vi "CounterStuff.vi"() -> ()   [LabVIEW 2012]
uses:
  <vilib>/DAQmx/write.llb/DAQmx Write (Analog 1D DBL 1Chan NSamp).vi
  <vilib>/DAQmx/create/channels.llb/DAQmx Create Channel (CO-Pulse Generation-Frequency).vi
  <vilib>/DAQmx/create/channels.llb/DAQmx Create Channel (AO-Voltage-Basic).vi
  <vilib>/DAQmx/configure/timing.llb/DAQmx Timing (Sample Clock).vi
  <vilib>/DAQmx/miscellaneous.llb/DAQmx Fill In Error Info.vi
panel:
  in  "stop":bool
  in  "Pixels (Lines)":dbl=256.0
  in  "Pixeltime (ms)":dbl=1.0
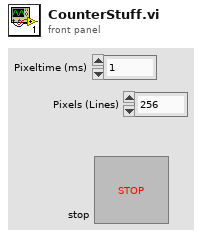
[diagram p1: front panel]
types:
  T1 = cluster{"task out":refnum<k21>, "task out":refnum<k21>, "task out":refnum<k21>, "task out":refnum<k21>}
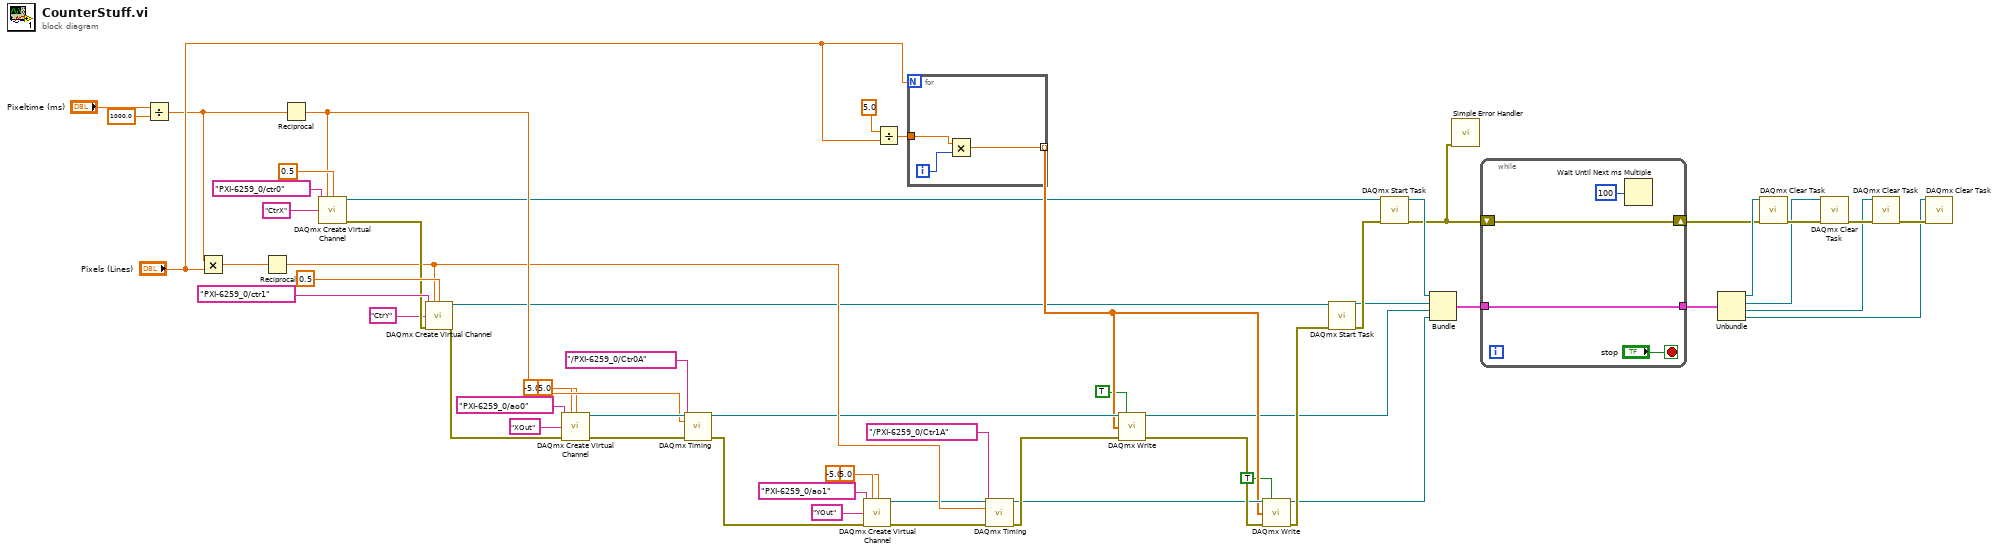
[diagram p0: block diagram]
diagram:
  n1 = Divide(x="Pixeltime (ms)", y=1000.0) -> (x/y=w7:dbl)
  n2 = Multiply(x=w7, y="Pixels (Lines)") -> (x*y=w55:dbl)
  n3 = Reciprocal(x=w55) -> (1/x=w42:dbl)
  n4 = Reciprocal(x=w7) -> (1/x=w47:dbl)
  n5 = call-poly <vilib>:"DAQmx Create Virtual Channel.vi"("frequency"=w47, "duty cycle"=0.5, "counter"=tag "PXI-6259_0/ctr0", "name to assign"="CtrX") -> ("task out"=w23:refnum<k21>, "error out"=w48:errorcluster)  [unwired: 10 in]
  n6 = call-poly <vilib>:"DAQmx Create Virtual Channel.vi"("frequency"=w42, "duty cycle"=0.5, "counter"=tag "PXI-6259_0/ctr1", "name to assign"="CtrY", "error in"=w48) -> ("task out"=w25:refnum<k21>, "error out"=w49:errorcluster)  [unwired: 9 in]
  n7 = call-poly <vilib>:"DAQmx Create Virtual Channel.vi"("maximum value"=5.0, "minimum value"=-5.0, "physical channels"=tag "PXI-6259_0/ao0", "name to assign"="XOut", "error in"=w49) -> ("task out"=w51:refnum<k21>, "error out"=w52:errorcluster)  [unwired: 9 in]
  n8 = call-poly <vilib>:"DAQmx Timing.vi"("task/channels in"=w51, "rate"=w47, "source"=tag "/PXI-6259_0/Ctr0A", "error in"=w52) -> ("task out"=w40:refnum<k21>, "error out"=w45:errorcluster)  [unwired: 10 in]
  n9 = call-poly <vilib>:"DAQmx Create Virtual Channel.vi"("maximum value"=5.0, "minimum value"=-5.0, "physical channels"=tag "PXI-6259_0/ao1", "name to assign"="YOut", "error in"=w45) -> ("task out"=w41:refnum<k21>, "error out"=w46:errorcluster)  [unwired: 9 in]
  n10 = Divide(x=5.0, y="Pixels (Lines)") -> (x/y=w30:dbl)
  n11 = for {
    N: "Pixels (Lines)" -> [_]
    tunnel: w30 -> [w61]
    tunnel: [w59] -> w29 mode=indexing
    i -> [w60]
    n12 = Multiply(x=w61, y=w60) -> (x*y=w59:dbl)
  }
  n13 = call-poly <vilib>:"DAQmx Timing.vi"("task/channels in"=w41, "rate"=w42, "source"=tag "/PXI-6259_0/Ctr1A", "error in"=w46) -> ("task out"=w37:refnum<k21>, "error out"=w39:errorcluster)  [unwired: 10 in]
  n14 = call-poly <vilib>:"DAQmx Write.vi"("task/channels in"=w40, "auto start"=TRUE, "data"=w29, "error in"=w39) -> ("task out"=w20:refnum<k21>, "error out"=w38:errorcluster)  [unwired: 9 in, 1 out]
  n15 = call-poly <vilib>:"DAQmx Write.vi"("task/channels in"=w37, "auto start"=TRUE, "data"=w29, "error in"=w38) -> ("task out"=w19:refnum<k21>, "error out"=w26:errorcluster)  [unwired: 9 in, 1 out]
  n16 = call <vilib>:"DAQmx Start Task.vi"("task/channels in"=w25, "error in"=w26) -> ("task out"=w21:refnum<k21>, "error out"=w24:errorcluster)  [unwired: 12 in]
  n17 = call <vilib>:"DAQmx Start Task.vi"("task/channels in"=w23, "error in"=w24) -> ("task out"=w22:refnum<k21>, "error out"=w5:errorcluster)  [unwired: 12 in]
  n18 = Bundle("task out"=w22, "task out"=w21, "task out"=w20, "task out"=w19) -> (w18:T1)  [unwired: 1 in]
  n19 = call <vilib>:"Simple Error Handler.vi"("error in (no error)"=w5) -> ()  [unwired: 4 in, 5 out]
  n20 = while {
    tunnel: w18 -> [w63]
    shift-right: [w64] -> w9
    shift-left: w5 -> [w64]
    tunnel: [w63] -> w17
    stop <- "stop" stop-if-true
    n21 = Wait Until Next ms Multiple(millisecond multiple=u32 100) -> ()  [unwired: 1 out]
  }
  n22 = Unbundle(w17) -> ("task out"=w16:refnum<k21>, "task out"=w14:refnum<k21>, "task out"=w12:refnum<k21>, "task out"=w10:refnum<k21>)
  n23 = call <vilib>:"DAQmx Clear Task.vi"("task in"=w16, "error in"=w9) -> ("error out"=w15:errorcluster)  [unwired: 13 in]
  n24 = call <vilib>:"DAQmx Clear Task.vi"("task in"=w14, "error in"=w15) -> ("error out"=w13:errorcluster)  [unwired: 13 in]
  n25 = call <vilib>:"DAQmx Clear Task.vi"("task in"=w12, "error in"=w13) -> ("error out"=w11:errorcluster)  [unwired: 13 in]
  n26 = call <vilib>:"DAQmx Clear Task.vi"("task in"=w10, "error in"=w11) -> ()  [unwired: 13 in, 1 out]
